vi "Carriage Intake Immediate.vi"(0 "Setpoint Left":dbl, 1 "Description":string, 5 "Extend":bool, 7 "Open":bool, 9 "Close":bool, 11 "Command Info In":T1, 12 "Setpoint Right":dbl, 13 "Synchronication":enum16{"Start", "Wait"}(ring)) -> (15 "Command Info Out":T1)   [LabVIEW 2018]
doc: "This template is useful for immediate subsystem actions that do not need deadband filtering\n\nBe sure to right-click and select New from Template and save with a new command name."
uses:
  <vilib>/Rock Robotics/WPI/Framework/Command Status Info.ctl
  <vilib>/Rock Robotics/WPI/Framework/Completion Status.ctl
  <vilib>/Rock Robotics/WPI/Framework/Completion Notifier.ctl
  Implementation/Carriage Intake Setpoints.ctl
  Implementation/Carriage Intake Operations.ctl
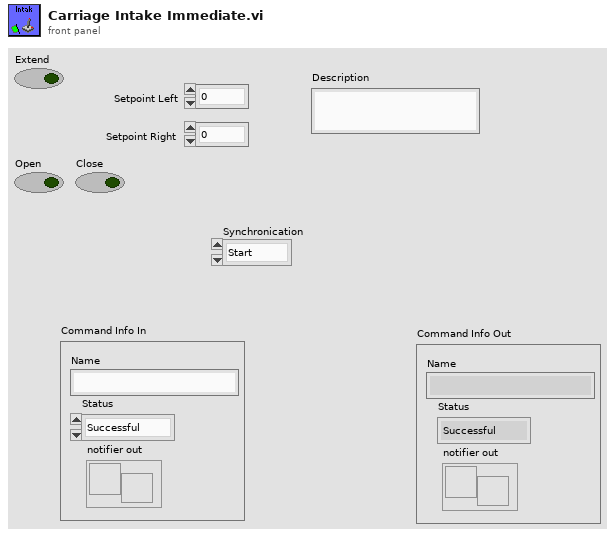
[diagram p1: front panel]
types:
  T1 = typedef "Command Status Info.ctl" = cluster{"Name":string, "Status":T2, "notifier out":T3}
  T2 = typedef "Completion Status.ctl" = enum16{"Successful", "Aborted", "Incomplete"}
  T3 = typedef "Completion Notifier.ctl" = refnum<notifier>
  T4 = typedef "Carriage Intake Setpoints.ctl" = cluster{"Operation":T5, "Left":dbl, "Duration":dbl, "Extend":bool, "Open":bool, "Close":bool, "Right":dbl}
  T5 = typedef "Carriage Intake Operations.ctl" = enum16{"Reserve", "Read Current", "Immediate"}
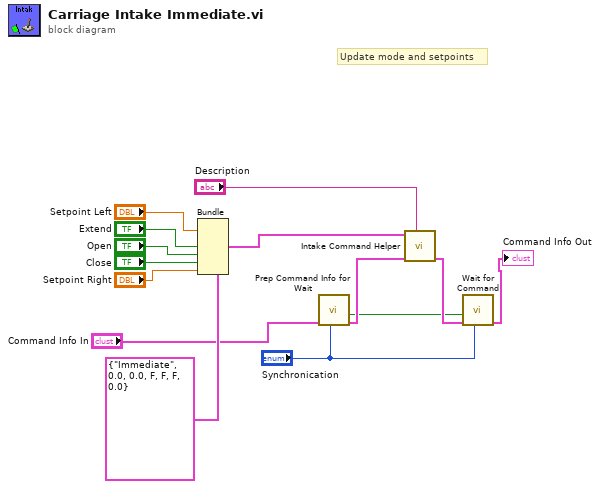
[diagram p0: block diagram]
diagram:
  # "Update mode and setpoints"
  n1 = Bundle(cluster=T4 {"Operation"=enum."Immediate", "Left"=0.0, "Duration"=0.0, "Extend"=FALSE, "Open"=FALSE, "Close"=FALSE, "Right"=0.0} ("SubSystem Data"), "Left"="Setpoint Left", "Extend"="Extend", "Open"="Open", "Close"="Close", "Right"="Setpoint Right") -> (w11:T4)  [unwired: 2 in]
  n2 = call <vilib>:"Prep Command Info for Wait.vi"("Synchronication"="Synchronication", "Command Info"="Command Info In") -> ("Command Info"=w4:T1, "Allocated"=w1:bool)  [unwired: 8 in]
  n3 = call "Intake Command Helper.vi"("Description"="Description", "Command Info In"=w4, "SubSystem Data"=w11) -> ("Command Info Out"=w3:T1)  [unwired: 6 in, 2 out]
  n4 = call <vilib>:"Wait for Command.vi"("Synchronication"="Synchronication", "Command Info in"=w3, "Allocated"=w1) -> ("Command Info out"=→"Command Info Out":T1)  [unwired: 8 in]
